vi "WPI_CameraSetModeAttr_EDIT.vi"(7 "Attr Format":string="CameraAttributes::%s::Mode", 8 "error in (no error)":errorcluster, 9 "Value":string="Manual", 10 "Attr String":string, 11 "Camera Address In":string) -> (0 "error out":errorcluster, 3 "Camera Address Out":string)   [LabVIEW 2015]
doc: "Set the Mode of the attribute to Manual or Auto.\n\nThis software is licensed. Open the labview\\readme\\WPI Robotics Library Open Source License.txt file for more information."
uses:
  <vilib>/userdefined/High Color/IMAQdx.ctl
  <resource>/objmgr/imaqdx.rc
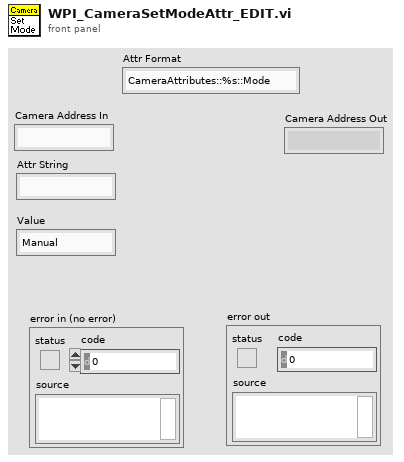
[diagram p1: front panel]
types:
  T1 = typedef "IMAQdx.ctl" = refnum<k21>
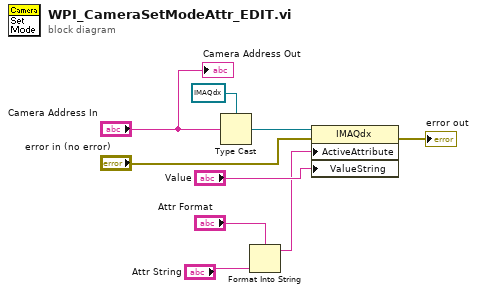
[diagram p0: block diagram]
diagram:
  n1 = Type Cast(type=T1 refnum ("Session In"), x="Camera Address In") -> (*(type *) &x=w7:T1)
  n2 = Format Into String(format string="Attr Format", "Attr String") -> (resulting string=w5:string)  [unwired: 2 in, 1 out]
  n3 = property class="IMAQdx"(reference=w7, error in="error in (no error)", "ActiveAttribute"=w5, "ValueString"="Value") -> (error out=→"error out":errorcluster)  [unwired: 1 out]
  "Camera Address Out" <- "Camera Address In"
